vi "传感器测试单片译码器.vi"() -> ()   [LabVIEW 2018]
panel:
  in  "Vot":dbl
  in  "reference resitance":dbl
  in  "File Name":string
  in  "File Path":path
  out "缓存 2":dbl
  out "缓存":dbl
  out "data 6":bool[](array[boolean]) caption="数据"
  out "初始化的数组 2":dbl[][](array[numeric])
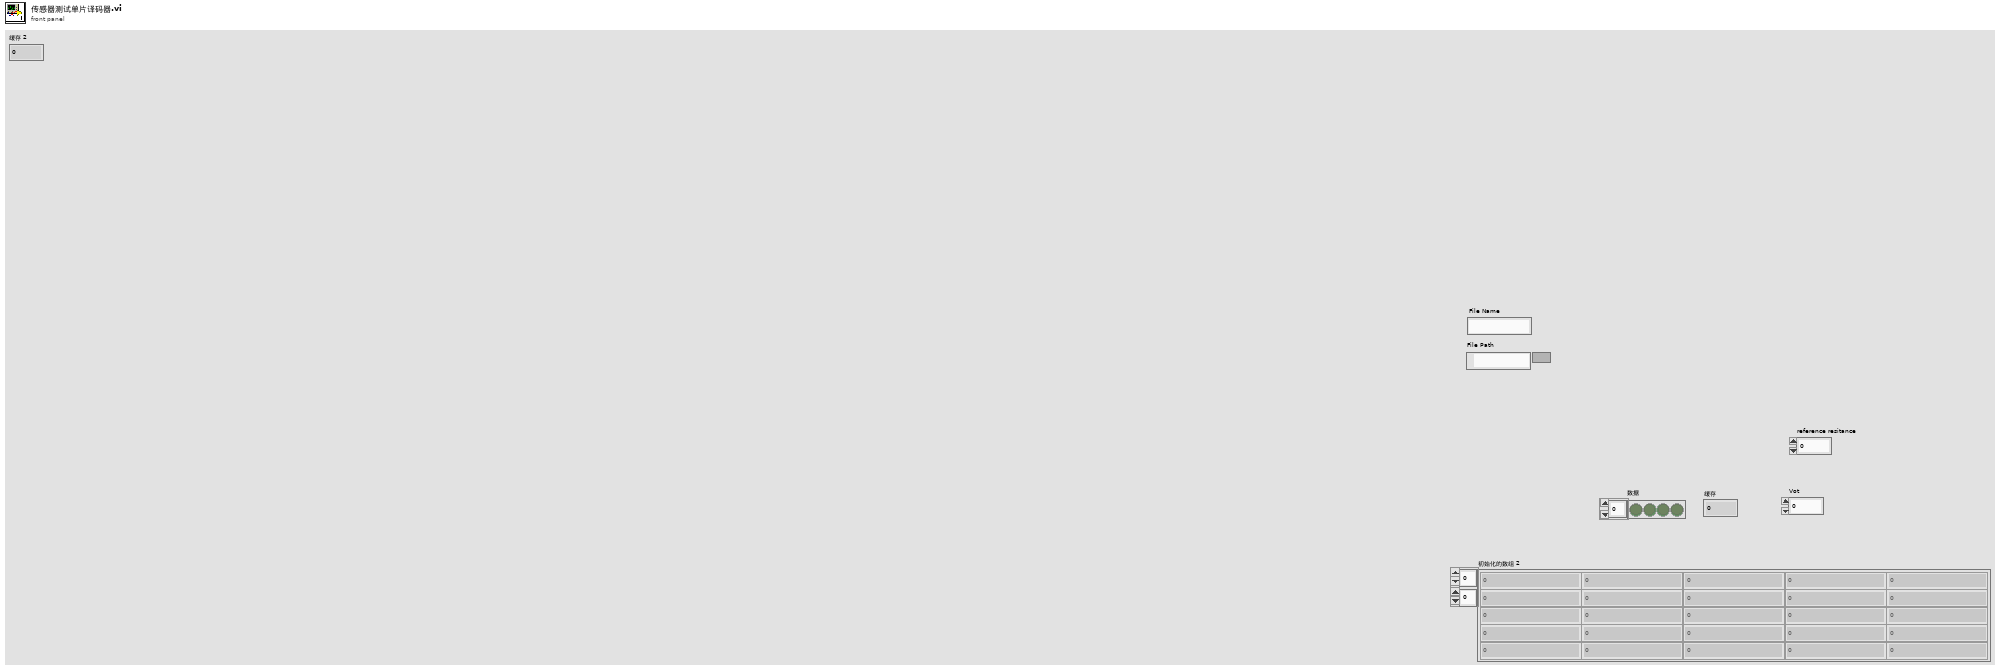
[diagram p1: front panel]
types:
  T1 = enum16{"open", "replace", "create", "open or create", "replace or create", "replace or create with confirmation"}
  T2 = enum16{"初始化", "s11", "s12", "s13", "s14", "s15", "s21", "s22", "s23", "s24", "s25", "s31", "s32", "s33", "s34", "s35"}
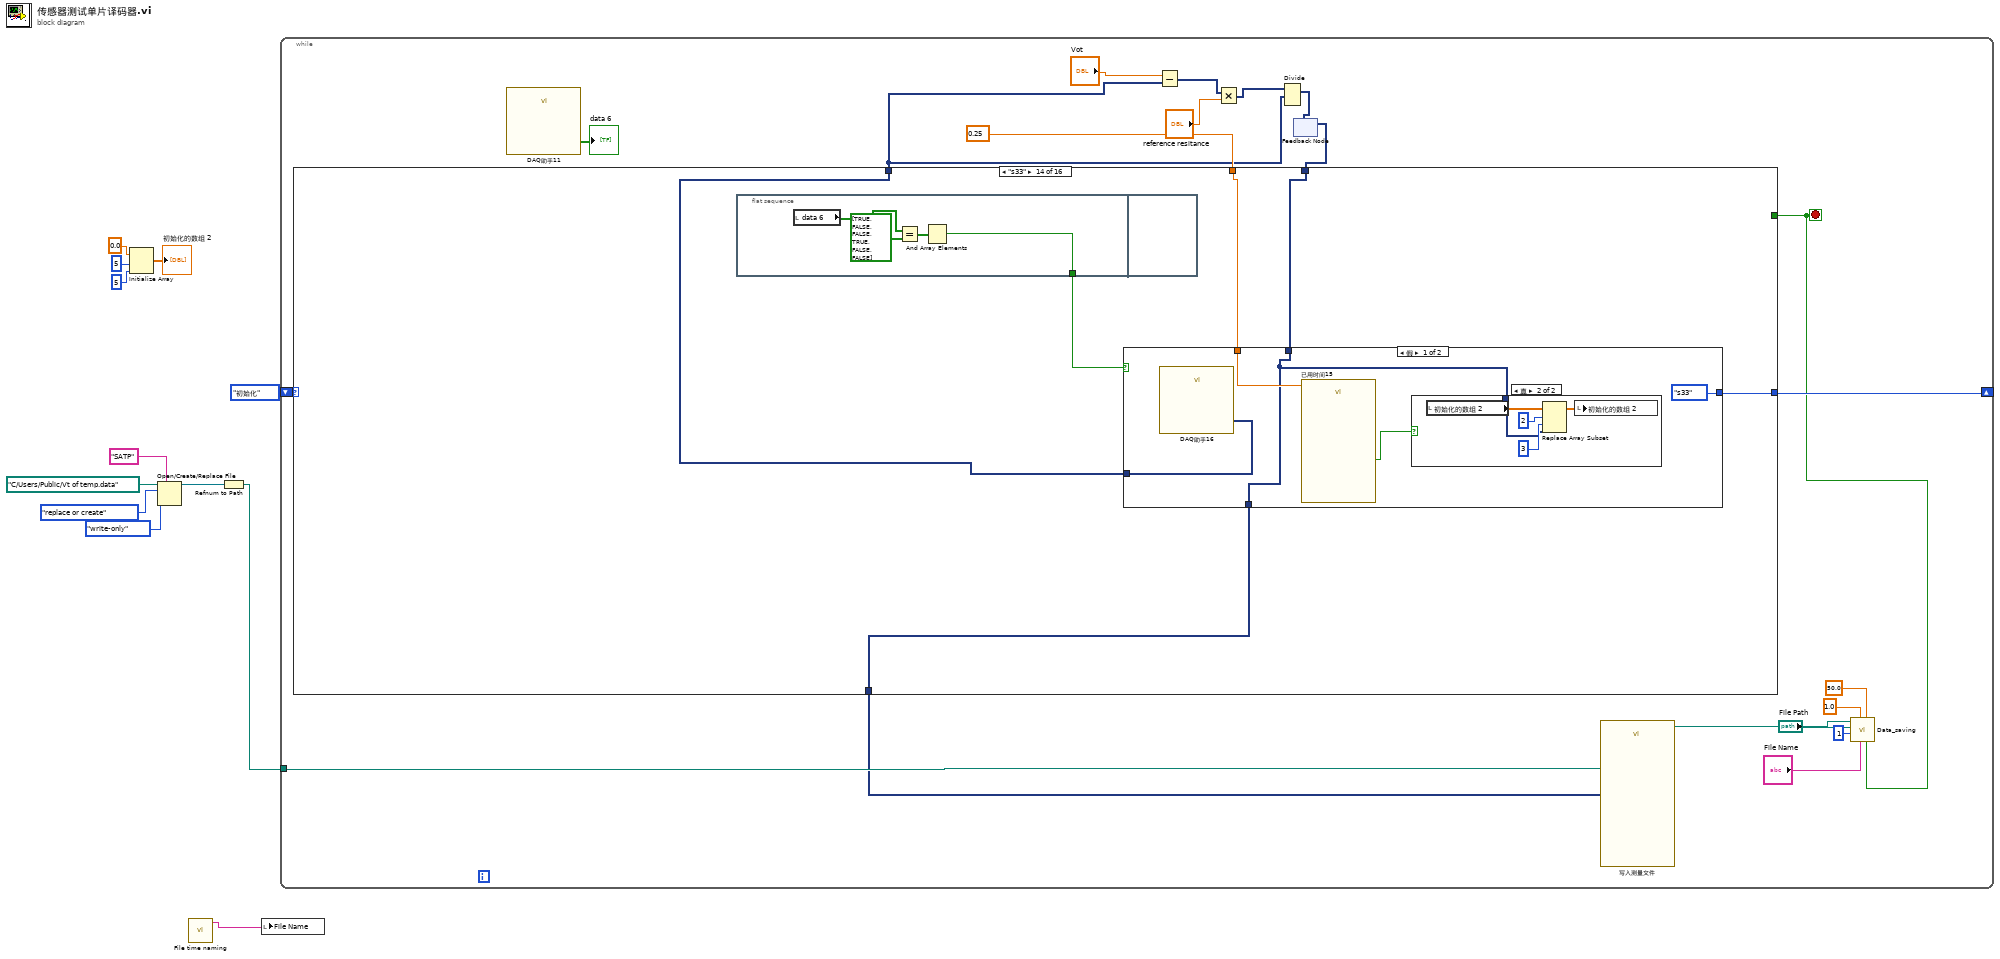
[diagram p0: block diagram]
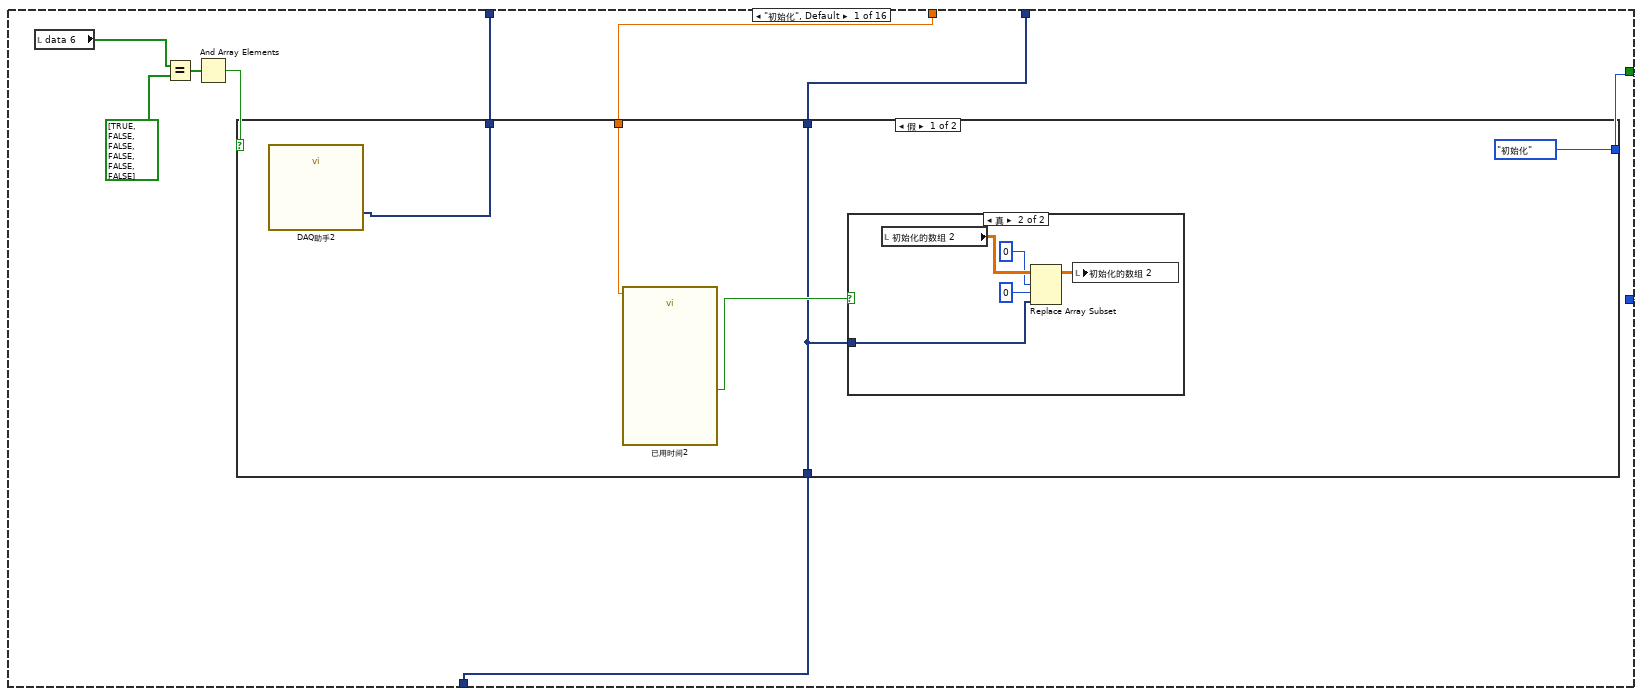
[diagram p2: hidden frame]
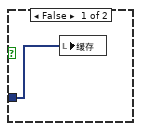
[diagram p3: hidden frame]
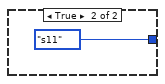
[diagram p4: hidden frame]
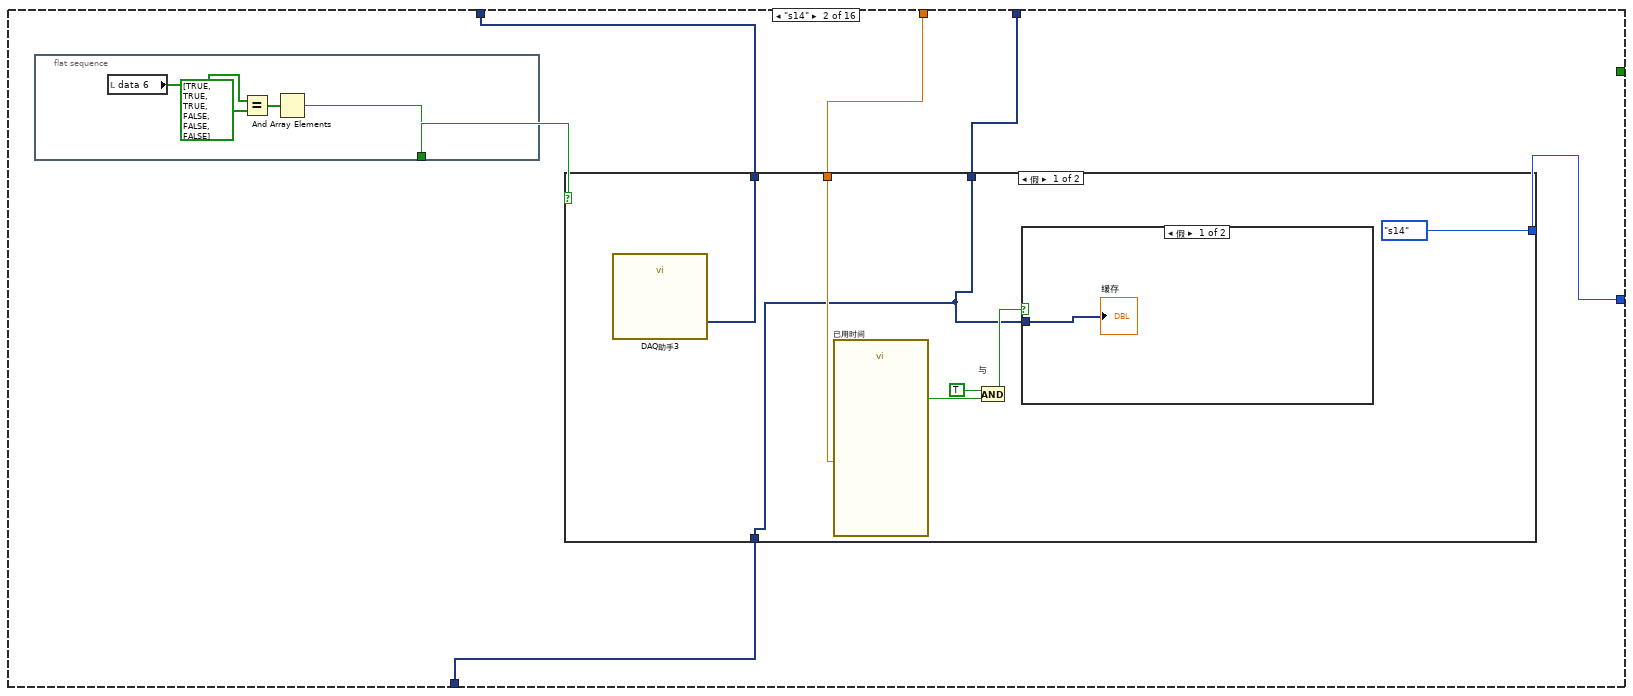
[diagram p5: hidden frame]
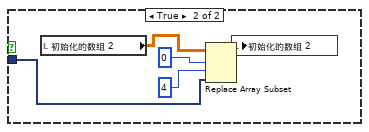
[diagram p6: hidden frame]
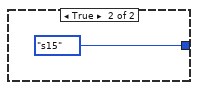
[diagram p7: hidden frame]
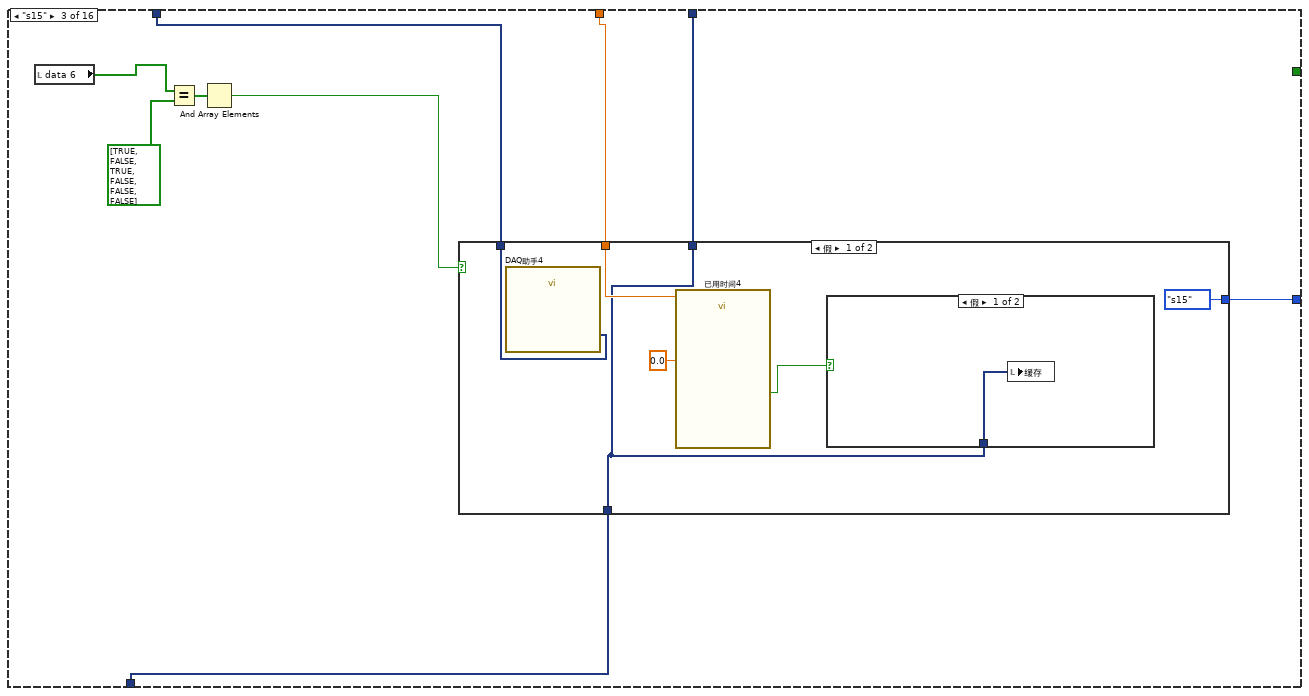
[diagram p8: hidden frame]
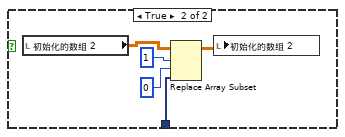
[diagram p9: hidden frame]
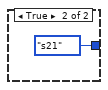
[diagram p10: hidden frame]
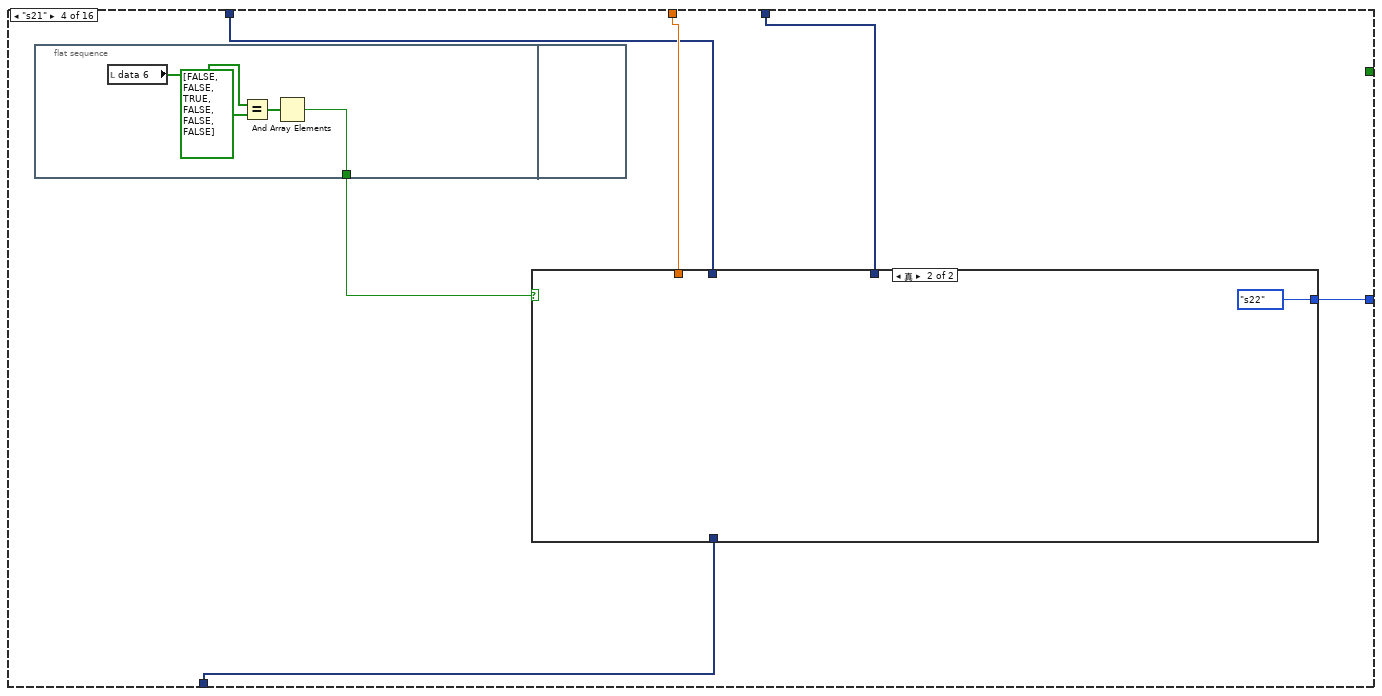
[diagram p11: hidden frame]
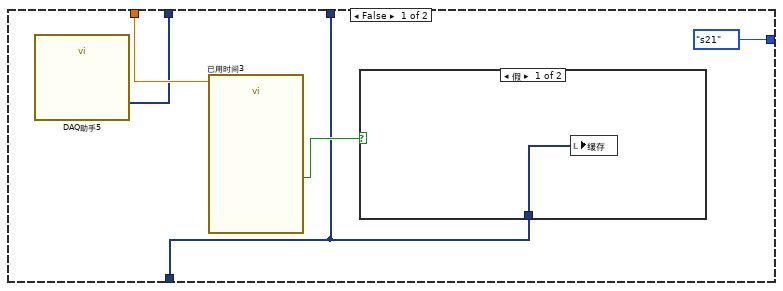
[diagram p12: hidden frame]
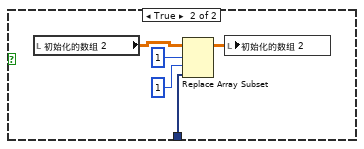
[diagram p13: hidden frame]
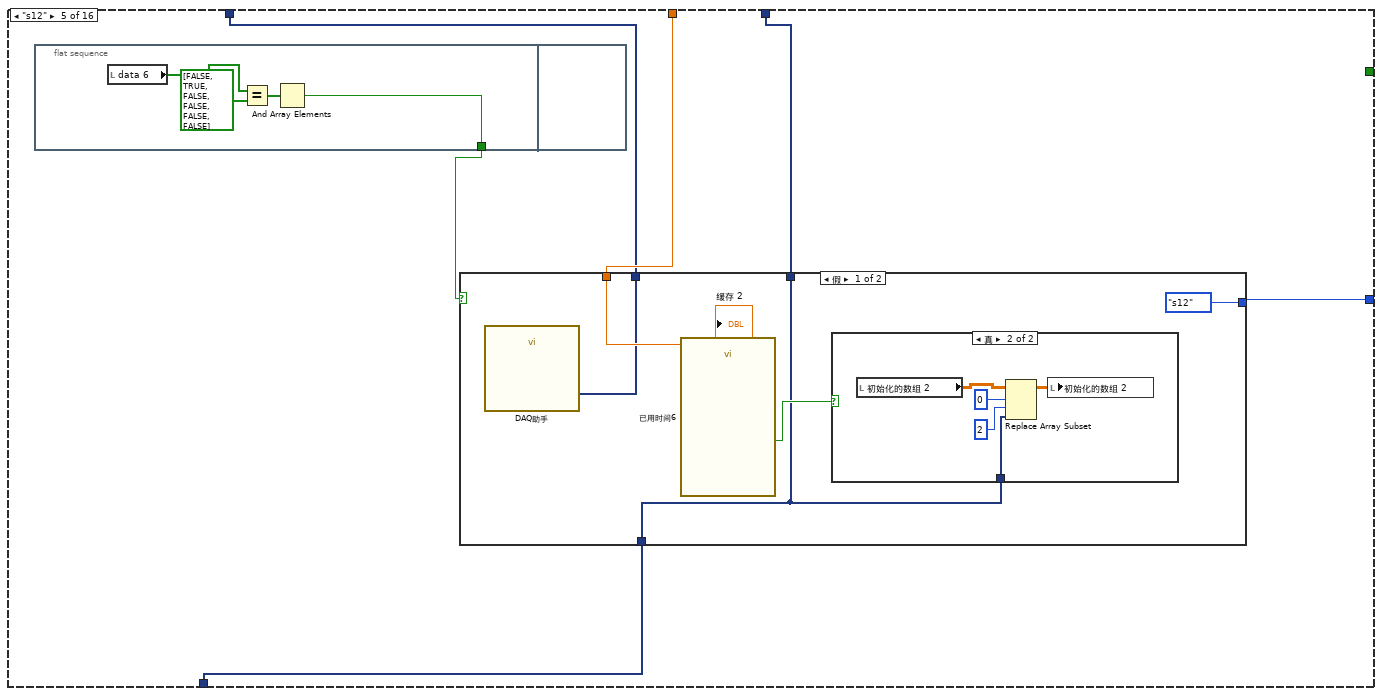
[diagram p14: hidden frame]
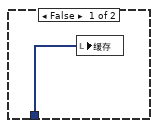
[diagram p15: hidden frame]
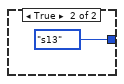
[diagram p16: hidden frame]
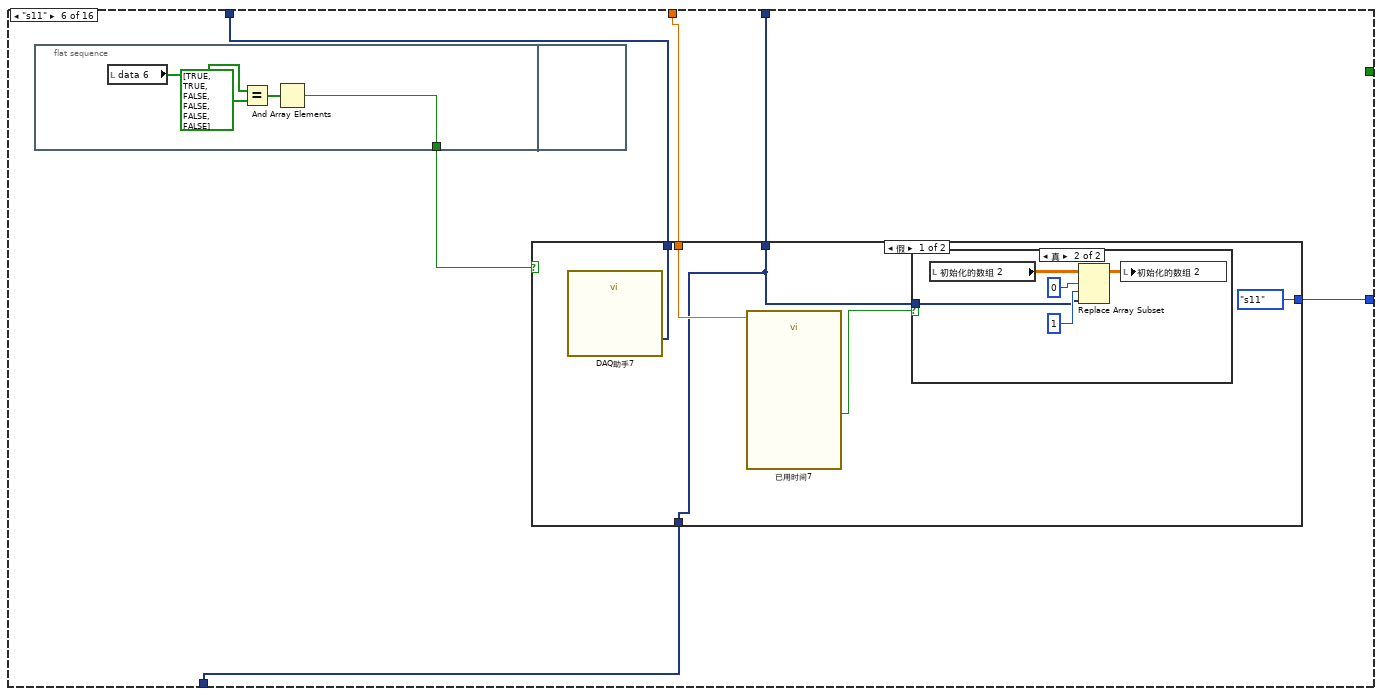
[diagram p17: hidden frame]
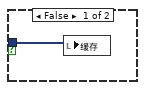
[diagram p18: hidden frame]
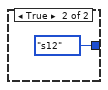
[diagram p19: hidden frame]
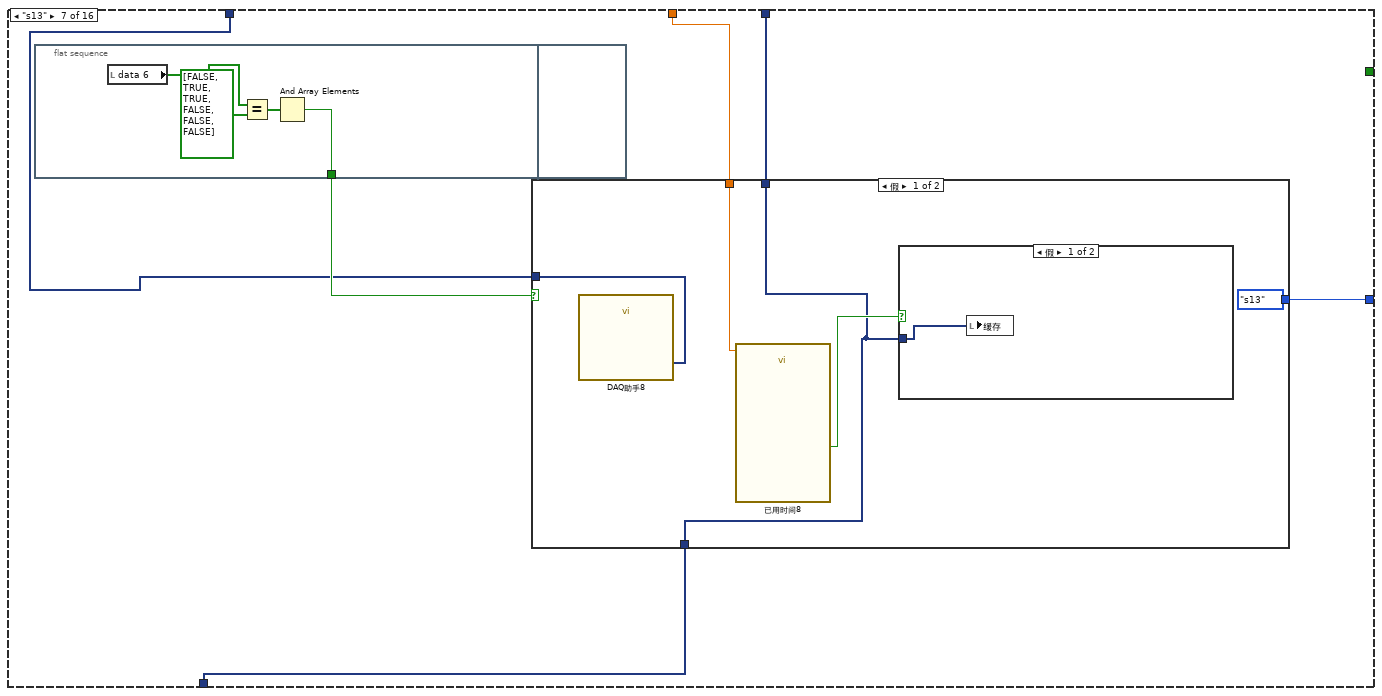
[diagram p20: hidden frame]
diagram:
  n1 = Initialize Array(0.0 ("元素"), 5 ("维数大小"), 5 ("维数大小")) -> (→"初始化的数组 2":dbl[][])
  n2 = Open/Create/Replace File(file path (use dialog)=path "C:/Users/Public/Vt of temp.data" ("文件路径（使用对话框）"), prompt="SATP" ("提示"), operation (0:open)=T1."replace or create" ("操作(0:open)"), access (0:read/write)=enum16{"read/write", "read-only", "write-only"}."write-only" ("权限(0:read/write)")) -> (refnum out=w4:refnum<file>)  [unwired: 2 in, 2 out]
  n3 = call "File time naming.vi"() -> ("result string"=w1:string)  [unwired: 11 in]
  n4 = Refnum to Path(1:w4) -> (0:w2:path)
  n5 = local write "File Name"(w1) -> ()
  n6 = while {
    shift-right: [w31] -> _
    shift-left: T2."初始化" ("枚举") -> [w32]
    tunnel: w2 -> [w28]
    stop <- w22 stop-if-true
    n7 = call "DAQ助手11"() -> ("data"=→"data 6":bool[])  [unwired: 17 in, 2 out]
    n8 = feedback #1() -> (w14:dynamicdata)  [unwired: 1 in]
    n9 = case shown="\"s33\"" w32 {
      tunnel: [w41 w59 w86 w105 w125 w149 w171 w193 w215 w237 w259 w281 w303 w325 w347 w369] -> w31
      tunnel: [_ _ _ _ _ _ _ _ _ _ _ _ _ _ _ w370] -> w22
      tunnel: 0.25 ("Time Target (s)") -> [w36 w57 w81 w103 w126 w147 w169 w191 w213 w235 w257 w279 w301 w323 w345 w367]
      tunnel: [w33 w56 w80 w102 w124 w146 w168 w190 w212 w234 w256 w278 w300 w322 w344 w366] -> w27
      tunnel: [w35 w55 w79 w101 w123 w145 w167 w189 w210 w233 w255 w276 w298 w321 w342 w364] -> w15
      tunnel: w14 -> [w34 w54 w78 w100 w122 w144 w166 w188 w211 w232 w254 w277 w299 w320 w343 w365]
      frame "初始化", Default {
        n10 = local read "data 6"() -> (w39:bool[])
        n11 = Equal?(x=w39, y=bool[] [TRUE, FALSE, FALSE, FALSE, FALSE, FALSE]) -> (x = y?=w40:bool[])
        n12 = And Array Elements(Boolean array=w40) -> (logical AND=w37:bool)
        n13 = case shown="假" w37 {
          tunnel: [T2."初始化" ("枚举") T2."s11" ("枚举")] -> w41
          tunnel: w36 -> [w45 _]
          tunnel: [w43 _] -> w35
          tunnel: w34 -> [w42 _]
          tunnel: [w42 _] -> w33
          frame False {
            n14 = call "DAQ助手2"() -> ("data"=w43:dynamicdata)  [unwired: 17 in, 2 out]
            n15 = call "已用时间2"("Time Target (s)"=w45) -> ("Time has Elapsed"=w44:bool)  [unwired: 11 in, 7 out]
            n16 = case shown="真" w44 {
              tunnel: w42 -> [w47 w48]
              frame False {
                n17 = local write "缓存"(w47) -> ()
              }
              frame True {
                n18 = local read "初始化的数组 2"() -> (w52:dbl[][])
                n19 = Replace Array Subset(array=w52, new element=w48, index (row)=0 ("禁用的索引 (行)"), index (col)=0 ("禁用的索引 (列)")) -> (w49:dbl[][])
                n20 = local write "初始化的数组 2"(w49) -> ()
              }
            }
          }
          frame True {
          }
        }
      }
      frame "s14" {
        n21 = flat-sequence {
          tunnel: [w60] -> w58
          frame #0 {
            n22 = local read "data 6"() -> (w63:bool[])
            n23 = Equal?(x=w63, y=bool[] [TRUE, TRUE, TRUE, FALSE, FALSE, FALSE]) -> (x = y?=w62:bool[])
            n24 = And Array Elements(Boolean array=w62) -> (logical AND=w60:bool)
          }
        }
        n25 = case shown="假" w58 {
          tunnel: [T2."s14" ("枚举") T2."s15" ("枚举")] -> w59
          tunnel: w57 -> [w66 _]
          tunnel: [w64 _] -> w56
          tunnel: [w65 _] -> w55
          tunnel: w54 -> [w64 _]
          frame False {
            n26 = call "DAQ助手3"() -> ("data"=w65:dynamicdata)  [unwired: 17 in, 2 out]
            n27 = call "已用时间"("Time Target (s)"=w66) -> ("Time has Elapsed"=w69:bool)  [unwired: 11 in, 7 out]
            n28 = And "与"(x=TRUE, y=w69) -> (x .and. y?=w68:bool)
            n29 = case shown="假" w68 {
              tunnel: w64 -> [w71 w72]
              frame False {
                "缓存" <- w71
              }
              frame True {
                n30 = local read "初始化的数组 2"() -> (w75:dbl[][])
                n31 = Replace Array Subset(array=w75, new element=w72, index (row)=0 ("禁用的索引 (行)"), index (col)=4 ("禁用的索引 (列)")) -> (w76:dbl[][])
                n32 = local write "初始化的数组 2"(w76) -> ()
              }
            }
          }
          frame True {
          }
        }
      }
      frame "s15" {
        n33 = local read "data 6"() -> (w84:bool[])
        n34 = Equal?(x=w84, y=bool[] [TRUE, FALSE, TRUE, FALSE, FALSE, FALSE]) -> (x = y?=w83:bool[])
        n35 = And Array Elements(Boolean array=w83) -> (logical AND=w85:bool)
        n36 = case shown="假" w85 {
          tunnel: [T2."s15" ("枚举") T2."s21" ("枚举")] -> w86
          tunnel: w81 -> [w91 _]
          tunnel: [w87 _] -> w80
          tunnel: [w88 _] -> w79
          tunnel: w78 -> [w87 _]
          frame False {
            n37 = call "DAQ助手4"() -> ("data"=w88:dynamicdata)  [unwired: 17 in, 2 out]
            n38 = call "已用时间4"("Time Target (s)"=w91, "Set Start Time (s)"=0.0) -> ("Time has Elapsed"=w89:bool)  [unwired: 10 in, 7 out]
            n39 = case shown="假" w89 {
              tunnel: w87 -> [w93 w94]
              frame False {
                n40 = local write "缓存"(w93) -> ()
              }
              frame True {
                n41 = local read "初始化的数组 2"() -> (w97:dbl[][])
                n42 = Replace Array Subset(array=w97, new element=w94, index (row)=1 ("禁用的索引 (行)"), index (col)=0 ("禁用的索引 (列)")) -> (w98:dbl[][])
                n43 = local write "初始化的数组 2"(w98) -> ()
              }
            }
          }
          frame True {
          }
        }
      }
      frame "s21" {
        n44 = flat-sequence {
          tunnel: [w106] -> w104
          frame #0 {
            n45 = local read "data 6"() -> (w109:bool[])
            n46 = Equal?(x=w109, y=bool[] [FALSE, FALSE, TRUE, FALSE, FALSE, FALSE]) -> (x = y?=w108:bool[])
            n47 = And Array Elements(Boolean array=w108) -> (logical AND=w106:bool)
          }
          frame #1 {
          }
        }
        n48 = case shown="真" w104 {
          tunnel: [T2."s21" ("枚举") T2."s22" ("枚举")] -> w105
          tunnel: w103 -> [w113 _]
          tunnel: [w110 _] -> w102
          tunnel: [w111 _] -> w101
          tunnel: w100 -> [w110 _]
          frame False {
            n49 = call "DAQ助手5"() -> ("data"=w111:dynamicdata)  [unwired: 17 in, 2 out]
            n50 = call "已用时间3"("Time Target (s)"=w113) -> ("Time has Elapsed"=w112:bool)  [unwired: 11 in, 7 out]
            n51 = case shown="假" w112 {
              tunnel: w110 -> [w115 w116]
              frame False {
                n52 = local write "缓存"(w115) -> ()
              }
              frame True {
                n53 = local read "初始化的数组 2"() -> (w119:dbl[][])
                n54 = Replace Array Subset(array=w119, new element=w116, index (row)=1 ("禁用的索引 (行)"), index (col)=1 ("禁用的索引 (列)")) -> (w120:dbl[][])
                n55 = local write "初始化的数组 2"(w120) -> ()
              }
            }
          }
          frame True {
          }
        }
      }
      frame "s12" {
        n56 = flat-sequence {
          tunnel: [w140] -> w127
          frame #0 {
            n57 = local read "data 6"() -> (w143:bool[])
            n58 = Equal?(x=w143, y=bool[] [FALSE, TRUE, FALSE, FALSE, FALSE, FALSE]) -> (x = y?=w142:bool[])
            n59 = And Array Elements(Boolean array=w142) -> (logical AND=w140:bool)
          }
          frame #1 {
          }
        }
        n60 = case shown="假" w127 {
          tunnel: [T2."s12" ("枚举") T2."s13" ("枚举")] -> w125
          tunnel: w126 -> [w131 _]
          tunnel: [w128 _] -> w124
          tunnel: [w129 _] -> w123
          tunnel: w122 -> [w128 _]
          frame False {
            n61 = call "DAQ助手"() -> ("data"=w129:dynamicdata)  [unwired: 17 in, 2 out]
            n62 = call "已用时间6"("Time Target (s)"=w131) -> ("Time has Elapsed"=w130:bool)  [unwired: 11 in, 7 out]
            n63 = case shown="真" w130 {
              tunnel: w128 -> [w133 w134]
              frame False {
                n64 = local write "缓存"(w133) -> ()
              }
              frame True {
                n65 = local read "初始化的数组 2"() -> (w137:dbl[][])
                n66 = Replace Array Subset(array=w137, new element=w134, index (row)=0 ("禁用的索引 (行)"), index (col)=2 ("禁用的索引 (列)")) -> (w138:dbl[][])
                n67 = local write "初始化的数组 2"(w138) -> ()
              }
            }
          }
          frame True {
          }
        }
      }
      frame "s11" {
        n68 = flat-sequence {
          tunnel: [w150] -> w148
          frame #0 {
            n69 = local read "data 6"() -> (w152:bool[])
            n70 = Equal?(x=w152, y=bool[] [TRUE, TRUE, FALSE, FALSE, FALSE, FALSE]) -> (x = y?=w153:bool[])
            n71 = And Array Elements(Boolean array=w153) -> (logical AND=w150:bool)
          }
          frame #1 {
          }
        }
        n72 = case shown="假" w148 {
          tunnel: [T2."s11" ("枚举") T2."s12" ("枚举")] -> w149
          tunnel: w147 -> [w157 _]
          tunnel: [w154 _] -> w146
          tunnel: [w155 _] -> w145
          tunnel: w144 -> [w154 _]
          frame False {
            n73 = call "DAQ助手7"() -> ("data"=w155:dynamicdata)  [unwired: 17 in, 2 out]
            n74 = call "已用时间7"("Time Target (s)"=w157) -> ("Time has Elapsed"=w156:bool)  [unwired: 11 in, 7 out]
            n75 = case shown="真" w156 {
              tunnel: w154 -> [w159 w160]
              frame False {
                n76 = local write "缓存"(w159) -> ()
              }
              frame True {
                n77 = local read "初始化的数组 2"() -> (w164:dbl[][])
                n78 = Replace Array Subset(array=w164, new element=w160, index (row)=0 ("禁用的索引 (行)"), index (col)=1 ("禁用的索引 (列)")) -> (w161:dbl[][])
                n79 = local write "初始化的数组 2"(w161) -> ()
              }
            }
          }
          frame True {
          }
        }
      }
      frame "s13" {
        n80 = flat-sequence {
          tunnel: [w172] -> w170
          frame #0 {
            n81 = local read "data 6"() -> (w175:bool[])
            n82 = Equal?(x=w175, y=bool[] [FALSE, TRUE, TRUE, FALSE, FALSE, FALSE]) -> (x = y?=w174:bool[])
            n83 = And Array Elements(Boolean array=w174) -> (logical AND=w172:bool)
          }
          frame #1 {
          }
        }
        n84 = case shown="假" w170 {
          tunnel: [T2."s13" ("枚举") T2."s14" ("枚举")] -> w171
          tunnel: w169 -> [w178 _]
          tunnel: [w176 _] -> w168
          tunnel: [w177 _] -> w167
          tunnel: w166 -> [w176 _]
          frame False {
            n85 = call "DAQ助手8"() -> ("data"=w177:dynamicdata)  [unwired: 17 in, 2 out]
            n86 = call "已用时间8"("Time Target (s)"=w178) -> ("Time has Elapsed"=w179:bool)  [unwired: 11 in, 7 out]
            n87 = case shown="假" w179 {
              tunnel: w176 -> [w181 w182]
              frame False {
                n88 = local write "缓存"(w181) -> ()
              }
              frame True {
                n89 = local read "初始化的数组 2"() -> (w185:dbl[][])
                n90 = Replace Array Subset(array=w185, new element=w182, index (row)=0 ("禁用的索引 (行)"), index (col)=3 ("禁用的索引 (列)")) -> (w186:dbl[][])
                n91 = local write "初始化的数组 2"(w186) -> ()
              }
            }
          }
          frame True {
          }
        }
      }
      frame "s22" {
        n92 = flat-sequence {
          tunnel: [w194] -> w192
          frame #0 {
            n93 = local read "data 6"() -> (w196:bool[])
            n94 = Equal?(x=w196, y=bool[] [FALSE, FALSE, TRUE, TRUE, FALSE, FALSE]) -> (x = y?=w197:bool[])
            n95 = And Array Elements(Boolean array=w197) -> (logical AND=w194:bool)
          }
          frame #1 {
          }
        }
        n96 = case shown="假" w192 {
          tunnel: [T2."s22" ("枚举") T2."s23" ("枚举")] -> w193
          tunnel: w191 -> [w201 _]
          tunnel: [w198 _] -> w190
          tunnel: [w199 _] -> w189
          tunnel: w188 -> [w198 _]
          frame False {
            n97 = call "DAQ助手9"() -> ("data"=w199:dynamicdata)  [unwired: 17 in, 2 out]
            n98 = call "已用时间9"("Time Target (s)"=w201) -> ("Time has Elapsed"=w200:bool)  [unwired: 11 in, 7 out]
            n99 = case shown="假" w200 {
              tunnel: w198 -> [w203 w204]
              frame False {
                n100 = local write "缓存"(w203) -> ()
              }
              frame True {
                n101 = local read "初始化的数组 2"() -> (w207:dbl[][])
                n102 = Replace Array Subset(array=w207, new element=w204, index (row)=1 ("禁用的索引 (行)"), index (col)=2 ("禁用的索引 (列)")) -> (w208:dbl[][])
                n103 = local write "初始化的数组 2"(w208) -> ()
              }
            }
          }
          frame True {
          }
        }
      }
      frame "s23" {
        n104 = flat-sequence {
          tunnel: [w216] -> w214
          frame #0 {
            n105 = local read "data 6"() -> (w218:bool[])
            n106 = Equal?(x=w218, y=bool[] [TRUE, FALSE, TRUE, TRUE, FALSE, FALSE]) -> (x = y?=w219:bool[])
            n107 = And Array Elements(Boolean array=w219) -> (logical AND=w216:bool)
          }
          frame #1 {
          }
        }
        n108 = case shown="假" w214 {
          tunnel: [T2."s23" ("枚举") T2."s24" ("枚举")] -> w215
          tunnel: w213 -> [w222 _]
          tunnel: [w221 _] -> w212
          tunnel: w211 -> [w221 _]
          tunnel: [w220 _] -> w210
          frame False {
            n109 = call "DAQ助手10"() -> ("data"=w220:dynamicdata)  [unwired: 17 in, 2 out]
            n110 = call "已用时间10"("Time Target (s)"=w222) -> ("Time has Elapsed"=w223:bool)  [unwired: 11 in, 7 out]
            n111 = case shown="真" w223 {
              tunnel: w221 -> [w225 w226]
              frame False {
                n112 = local write "缓存"(w225) -> ()
              }
              frame True {
                n113 = local read "初始化的数组 2"() -> (w229:dbl[][])
                n114 = Replace Array Subset(array=w229, new element=w226, index (row)=1 ("禁用的索引 (行)"), index (col)=3 ("禁用的索引 (列)")) -> (w230:dbl[][])
                n115 = local write "初始化的数组 2"(w230) -> ()
              }
            }
          }
          frame True {
          }
        }
      }
      frame "s24" {
        n116 = flat-sequence {
          tunnel: [w238] -> w236
          frame #0 {
            n117 = local read "data 6"() -> (w240:bool[])
            n118 = Equal?(x=w240, y=bool[] [TRUE, TRUE, TRUE, TRUE, FALSE, FALSE]) -> (x = y?=w241:bool[])
            n119 = And Array Elements(Boolean array=w241) -> (logical AND=w238:bool)
          }
          frame #1 {
          }
        }
        n120 = case shown="真" w236 {
          tunnel: [T2."s24" ("枚举") T2."s25" ("枚举")] -> w237
          tunnel: w235 -> [w244 _]
          tunnel: [w242 _] -> w234
          tunnel: [w243 _] -> w233
          tunnel: w232 -> [w242 _]
          frame False {
            n121 = call "DAQ助手12"() -> ("data"=w243:dynamicdata)  [unwired: 17 in, 2 out]
            n122 = call "已用时间11"("Time Target (s)"=w244) -> ("Time has Elapsed"=w245:bool)  [unwired: 11 in, 7 out]
            n123 = case shown="假" w245 {
              tunnel: w242 -> [w247 w248]
              frame False {
                n124 = local write "缓存"(w247) -> ()
              }
              frame True {
                n125 = local read "初始化的数组 2"() -> (w250:dbl[][])
                n126 = Replace Array Subset(array=w250, new element=w248, index (row)=1 ("禁用的索引 (行)"), index (col)=4 ("禁用的索引 (列)")) -> (w249:dbl[][])
                n127 = local write "初始化的数组 2"(w249) -> ()
              }
            }
          }
          frame True {
          }
        }
      }
      frame "s25" {
        n128 = flat-sequence {
          tunnel: [w260] -> w258
          frame #0 {
            n129 = local read "data 6"() -> (w262:bool[])
            n130 = Equal?(x=w262, y=bool[] [FALSE, TRUE, TRUE, TRUE, FALSE, FALSE]) -> (x = y?=w263:bool[])
            n131 = And Array Elements(Boolean array=w263) -> (logical AND=w260:bool)
          }
          frame #1 {
          }
        }
        n132 = case shown="真" w258 {
          tunnel: [T2."s25" ("枚举") T2."s31" ("枚举")] -> w259
          tunnel: w257 -> [w267 _]
          tunnel: [w264 _] -> w256
          tunnel: [w265 _] -> w255
          tunnel: w254 -> [w264 _]
          frame False {
            n133 = call "DAQ助手13"() -> ("data"=w265:dynamicdata)  [unwired: 17 in, 2 out]
            n134 = call "已用时间12"("Time Target (s)"=w267) -> ("Time has Elapsed"=w266:bool)  [unwired: 11 in, 7 out]
            n135 = case shown="假" w266 {
              tunnel: w264 -> [w269 w270]
              frame False {
                n136 = local write "缓存"(w269) -> ()
              }
              frame True {
                n137 = local read "初始化的数组 2"() -> (w272:dbl[][])
                n138 = Replace Array Subset(array=w272, new element=w270, index (row)=2 ("禁用的索引 (行)"), index (col)=0 ("禁用的索引 (列)")) -> (w271:dbl[][])
                n139 = local write "初始化的数组 2"(w271) -> ()
              }
            }
          }
          frame True {
          }
        }
      }
      frame "s31" {
        n140 = flat-sequence {
          tunnel: [w282] -> w280
          frame #0 {
            n141 = local read "data 6"() -> (w284:bool[])
            n142 = Equal?(x=w284, y=bool[] [FALSE, TRUE, FALSE, TRUE, FALSE, FALSE]) -> (x = y?=w285:bool[])
            n143 = And Array Elements(Boolean array=w285) -> (logical AND=w282:bool)
          }
          frame #1 {
          }
        }
        n144 = case shown="真" w280 {
          tunnel: [T2."s31" ("枚举") T2."s32" ("枚举")] -> w281
          tunnel: w279 -> [w289 _]
          tunnel: [w287 _] -> w278
          tunnel: w277 -> [w287 _]
          tunnel: [w286 _] -> w276
          frame False {
            n145 = call "DAQ助手14"() -> ("data"=w286:dynamicdata)  [unwired: 17 in, 2 out]
            n146 = call "已用时间13"("Time Target (s)"=w289) -> ("Time has Elapsed"=w288:bool)  [unwired: 11 in, 7 out]
            n147 = case shown="假" w288 {
              tunnel: w287 -> [w291 w292]
              frame False {
                n148 = local write "缓存"(w291) -> ()
              }
              frame True {
                n149 = local read "初始化的数组 2"() -> (w294:dbl[][])
                n150 = Replace Array Subset(array=w294, new element=w292, index (row)=2 ("禁用的索引 (行)"), index (col)=1 ("禁用的索引 (列)")) -> (w293:dbl[][])
                n151 = local write "初始化的数组 2"(w293) -> ()
              }
            }
          }
          frame True {
          }
        }
      }
      frame "s32" {
        n152 = flat-sequence {
          tunnel: [w304] -> w302
          frame #0 {
            n153 = local read "data 6"() -> (w306:bool[])
            n154 = Equal?(x=w306, y=bool[] [TRUE, TRUE, FALSE, TRUE, FALSE, FALSE]) -> (x = y?=w307:bool[])
            n155 = And Array Elements(Boolean array=w307) -> (logical AND=w304:bool)
          }
          frame #1 {
          }
        }
        n156 = case shown="真" w302 {
          tunnel: [T2."s32" ("枚举") T2."s33" ("枚举")] -> w303
          tunnel: w301 -> [w311 _]
          tunnel: [w309 _] -> w300
          tunnel: w299 -> [w309 _]
          tunnel: [w308 _] -> w298
          frame False {
            n157 = call "DAQ助手15"() -> ("data"=w308:dynamicdata)  [unwired: 17 in, 2 out]
            n158 = call "已用时间14"("Time Target (s)"=w311) -> ("Time has Elapsed"=w310:bool)  [unwired: 11 in, 7 out]
            n159 = case shown="假" w310 {
              tunnel: w309 -> [w313 w314]
              frame False {
                n160 = local write "缓存"(w313) -> ()
              }
              frame True {
                n161 = local read "初始化的数组 2"() -> (w316:dbl[][])
                n162 = Replace Array Subset(array=w316, new element=w314, index (row)=2 ("禁用的索引 (行)"), index (col)=2 ("禁用的索引 (列)")) -> (w315:dbl[][])
                n163 = local write "初始化的数组 2"(w315) -> ()
              }
            }
          }
          frame True {
          }
        }
      }
      frame "s33" {
        n164 = flat-sequence {
          tunnel: [w326] -> w324
          frame #0 {
            n165 = local read "data 6"() -> (w328:bool[])
            n166 = Equal?(x=w328, y=bool[] [TRUE, FALSE, FALSE, TRUE, FALSE, FALSE]) -> (x = y?=w329:bool[])
            n167 = And Array Elements(Boolean array=w329) -> (logical AND=w326:bool)
          }
          frame #1 {
          }
        }
        n168 = case shown="假" w324 {
          tunnel: [T2."s33" ("枚举") T2."s34" ("枚举")] -> w325
          tunnel: w323 -> [w333 _]
          tunnel: [w330 _] -> w322
          tunnel: [w331 _] -> w321
          tunnel: w320 -> [w330 _]
          frame False {
            n169 = call "DAQ助手16"() -> ("data"=w331:dynamicdata)  [unwired: 17 in, 2 out]
            n170 = call "已用时间15"("Time Target (s)"=w333) -> ("Time has Elapsed"=w332:bool)  [unwired: 11 in, 7 out]
            n171 = case shown="真" w332 {
              tunnel: w330 -> [w335 w336]
              frame False {
                n172 = local write "缓存"(w335) -> ()
              }
              frame True {
                n173 = local read "初始化的数组 2"() -> (w338:dbl[][])
                n174 = Replace Array Subset(array=w338, new element=w336, index (row)=2 ("禁用的索引 (行)"), index (col)=3 ("禁用的索引 (列)")) -> (w337:dbl[][])
                n175 = local write "初始化的数组 2"(w337) -> ()
              }
            }
          }
          frame True {
          }
        }
      }
      frame "s34" {
        n176 = flat-sequence {
          tunnel: [w348] -> w346
          frame #0 {
            n177 = local read "data 6"() -> (w350:bool[])
            n178 = Equal?(x=w350, y=bool[] [FALSE, FALSE, FALSE, TRUE, FALSE, FALSE]) -> (x = y?=w351:bool[])
            n179 = And Array Elements(Boolean array=w351) -> (logical AND=w348:bool)
          }
          frame #1 {
          }
        }
        n180 = case shown="真" w346 {
          tunnel: [T2."s34" ("枚举") T2."s35" ("枚举")] -> w347
          tunnel: w345 -> [w354 _]
          tunnel: [w352 _] -> w344
          tunnel: w343 -> [w352 _]
          tunnel: [w353 _] -> w342
          frame False {
            n181 = call "DAQ助手17"() -> ("data"=w353:dynamicdata)  [unwired: 17 in, 2 out]
            n182 = call "已用时间16"("Time Target (s)"=w354) -> ("Time has Elapsed"=w355:bool)  [unwired: 11 in, 7 out]
            n183 = case shown="真" w355 {
              tunnel: w352 -> [w357 w358]
              frame False {
                n184 = local write "缓存"(w357) -> ()
              }
              frame True {
                n185 = local read "初始化的数组 2"() -> (w360:dbl[][])
                n186 = Replace Array Subset(array=w360, new element=w358, index (row)=2 ("禁用的索引 (行)"), index (col)=4 ("禁用的索引 (列)")) -> (w359:dbl[][])
                n187 = local write "初始化的数组 2"(w359) -> ()
              }
            }
          }
          frame True {
          }
        }
      }
      frame "s35" {
        n188 = flat-sequence {
          tunnel: [w371] -> w368
          frame #0 {
            n189 = local read "data 6"() -> (w374:bool[])
            n190 = Equal?(x=w374, y=bool[] [FALSE, FALSE, FALSE, FALSE, FALSE, FALSE]) -> (x = y?=w372:bool[])
            n191 = And Array Elements(Boolean array=w372) -> (logical AND=w371:bool)
          }
        }
        n192 = case shown="真" w368 {
          tunnel: [_ TRUE] -> w370
          tunnel: [T2."s35" ("枚举") T2."s35" ("枚举")] -> w369
          tunnel: w367 -> [w378 _]
          tunnel: [w376 _] -> w366
          tunnel: w365 -> [w376 _]
          tunnel: [w375 _] -> w364
          frame False {
            n193 = call "DAQ助手18"() -> ("data"=w375:dynamicdata)  [unwired: 17 in, 2 out]
            n194 = call "已用时间5"("Time Target (s)"=w378) -> ("Time has Elapsed"=w377:bool)  [unwired: 11 in, 7 out]
            n195 = case shown="假" w377 {
              tunnel: w376 -> [w380 w381]
              frame False {
                n196 = local write "缓存"(w380) -> ()
              }
              frame True {
                n197 = local read "初始化的数组 2"() -> (w383:dbl[][])
                n198 = Replace Array Subset(array=w383, new element=w381, index (row)=3 ("禁用的索引 (行)"), index (col)=0 ("禁用的索引 (列)")) -> (w382:dbl[][])
                n199 = local write "初始化的数组 2"(w382) -> ()
              }
            }
          }
          frame True {
          }
        }
      }
    }
    n200 = Subtract(x="Vot", y=w15) -> (x-y=w17:dynamicdata)
    n201 = Multiply(x=w17, y="reference resitance") -> (x*y=w19:dynamicdata)
    n202 = Divide(1:w15, 2:w19) -> (0:w13:dynamicdata)  [unwired: 1 in, 1 out]
    n203 = feedback-in #1(w13) -> ()
    n204 = call "写入测量文件"("Signals"=w27, "Filename"=w28) -> ("Filename Out"=w20:path)  [unwired: 15 in, 2 out]
    n205 = call "Data_saving.vi"("Boolean"=w22, "Sampling Rate"=50.0, "File Name"="File Name", "Voltage Sensitivity\n1000 will be 1000"=1.0 ("Voltage Sensitivity\n1000 will be 1000"), "Number of Samples Per Channel"=1, "File Path"="File Path", "File name source"=w20) -> ()  [unwired: 5 in]
  }
